vi "GetTriggerSource.vi"(8 "Error In":errorcluster, 11 "Keithley 6482 In":refnum<visa-resource-name>) -> (0 "Error Out":errorcluster, 2 "Trigger Source":T1, 3 "Keithley 6482 Out":refnum<visa-resource-name>)   [LabVIEW 2012, in "Keithley-6482.lvlib"]
uses:
  Keithley-6482.lvlib
  Controls/TriggerSource.ctl
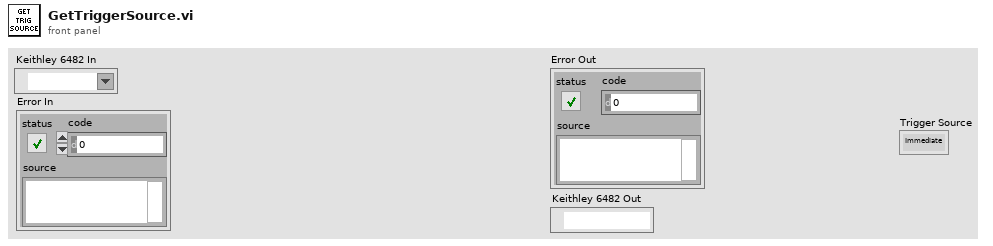
[diagram p1: front panel]
types:
  T1 = typedef "Keithley-6482.lvlib/TriggerSource.ctl" = enum16{"Immediate", "TLink"}
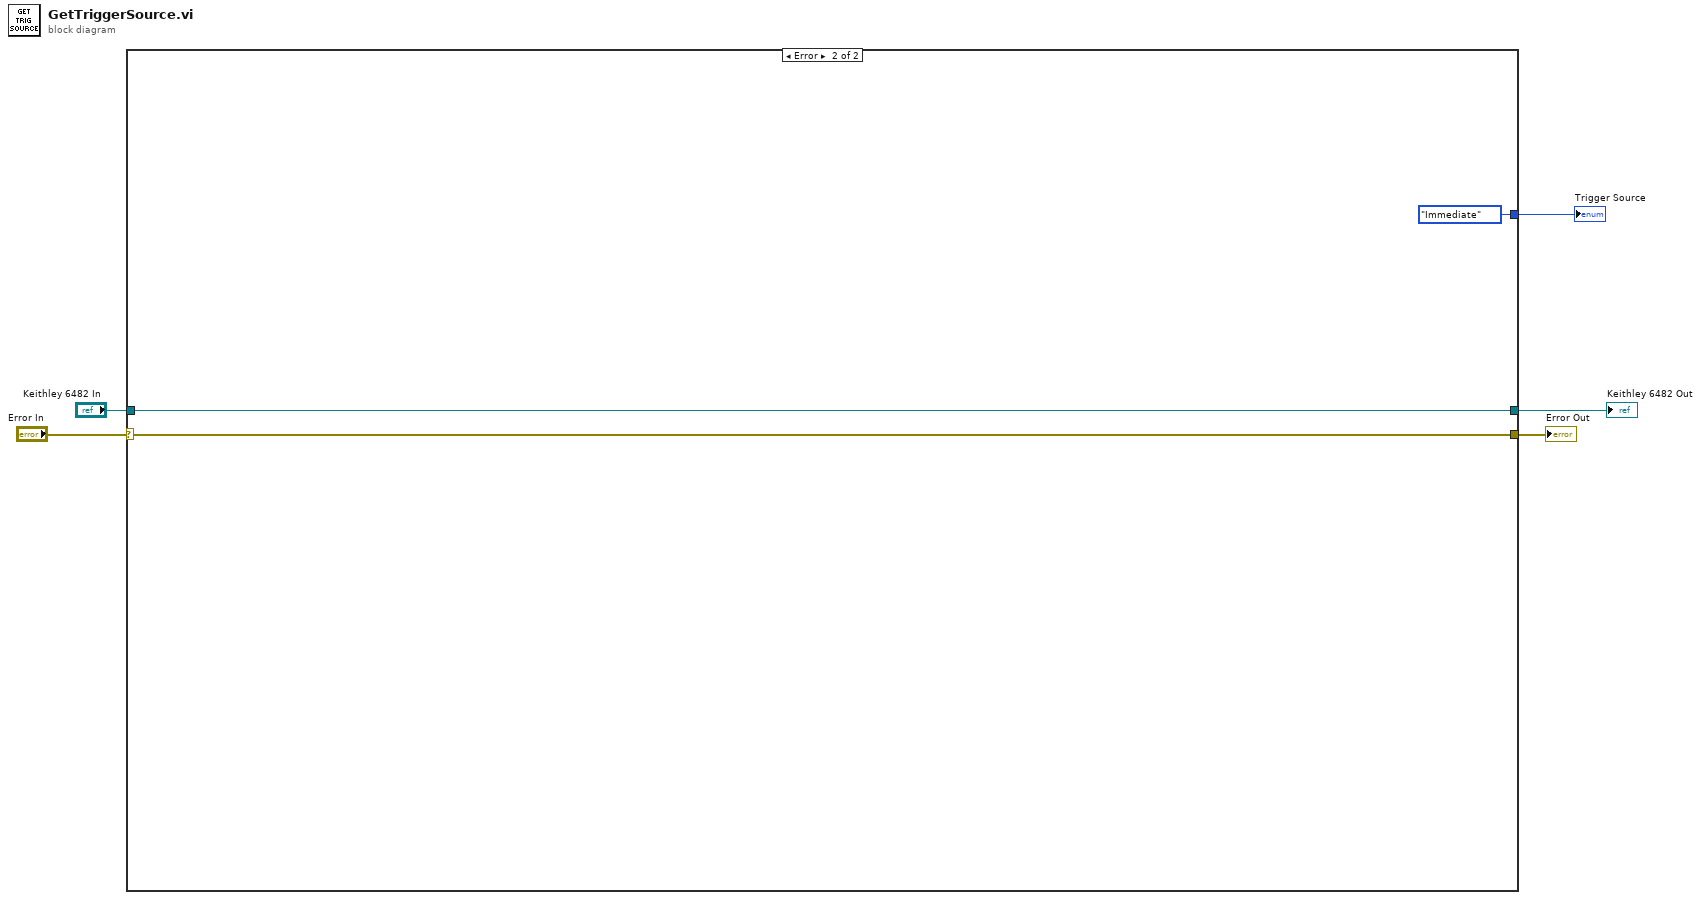
[diagram p0: block diagram]
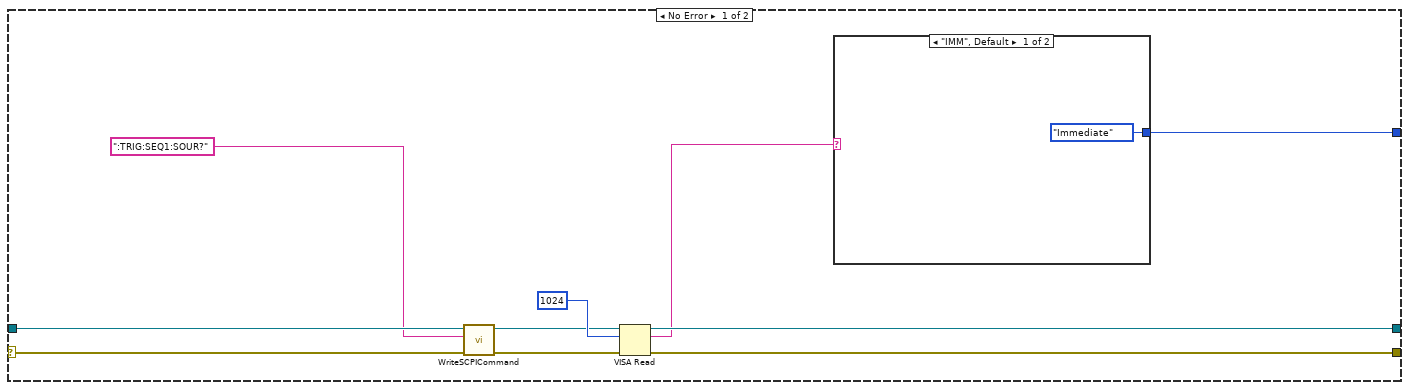
[diagram p2: hidden frame]
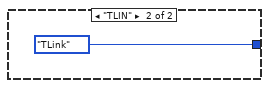
[diagram p3: hidden frame]
diagram:
  n1 = case shown="Error" "Error In" {
    selector: "Error In" -> [w10 w19]
    tunnel: "Keithley 6482 In" -> [w9 w20]
    tunnel: [w15 w19] -> w3
    tunnel: [w14 w20] -> w2
    tunnel: [w6 TriggerSource."Immediate" ("Trigger Source")] -> w1
    frame No Error {
      n2 = call "WriteSCPICommand.vi"("Error In"=w10, "SCPI Command"=":TRIG:SEQ1:SOUR?" ("string"), "Keithley 6482 In"=w9) -> ("Error Out"=w11:errorcluster, "Keithley 6482 Out"=w12:refnum<visa-resource-name>)  [unwired: 7 in]
      n3 = VISA Read(VISA resource name=w12, byte count=u32 1024, error in (no error)=w11) -> (VISA resource name out=w14:refnum<visa-resource-name>, read buffer=w7:string, error out=w15:errorcluster)  [unwired: 1 out]
      n4 = case shown="\"IMM\", Default" w7 {
        tunnel: [TriggerSource."Immediate" ("Trigger Source") TriggerSource."TLink" ("Trigger Source")] -> w6
        frame "IMM", Default {
        }
        frame "TLIN" {
        }
      }
    }
    frame Error {
    }
  }
  "Error Out" <- w3
  "Keithley 6482 Out" <- w2
  "Trigger Source" <- w1
